vi "CommsTests.vi"() -> (2 "Pressure(hPa)":dbl format="%.1f")   [LabVIEW 2018]
uses:
  <vilib>/httpClient/LabVIEWHTTPClient.lvlib
panel:
  in  "timeout ms (60000)":i32=2000
  out "error out 2":errorcluster
  in  "remote port or service name":u16=2000
  in  "address":string="10.245.87.30"
  in  "data in":string="*SRHb\n"
  out "data out":string
  out "error out":errorcluster
  out "body":string
  out "headers":string="\r\n"
  in  "url":string="http://192.168.126.101"
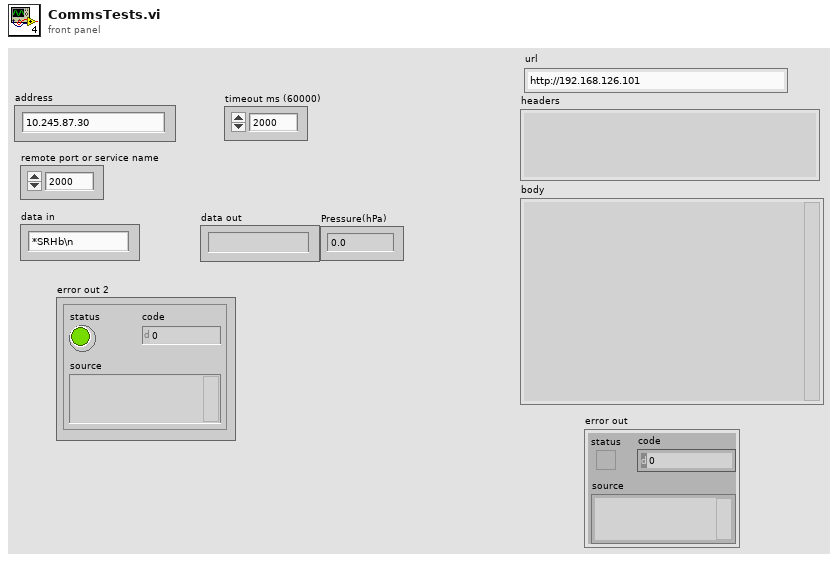
[diagram p1: front panel]
types:
  T1 = enum16{"Standard", "Buffered", "CRLF", "Immediate"}
  T2 = typedef "LabVIEWHTTPClient.lvlib/ClientHandle.ctl" = refnum<k1>
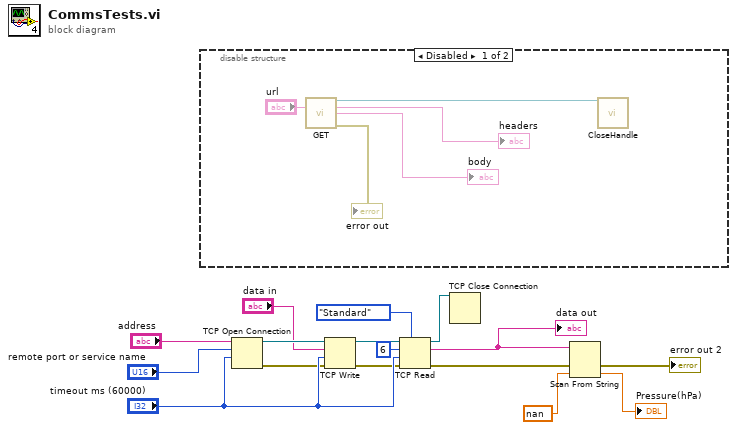
[diagram p0: block diagram]
diagram:
  n1 = disable-structure shown="Disabled" {
    frame Disabled {
      n2 = call <vilib>:"GET.vi"("url"="url") -> ("client handle out"=w17:T2, "headers"=→"headers":string, "body"=→"body":string, "error out"=→"error out":errorcluster)  [unwired: 11 in]
      n3 = call <vilib>:"CloseHandle.vi"("client handle"=w17) -> ()  [unwired: 14 in, 1 out]
    }
    frame Enabled {
    }
  }
  n4 = TCP Open Connection(address="address", remote port or service name="remote port or service name", timeout ms (60000)="timeout ms (60000)") -> (connection ID=w16:refnum<k5>, error out=w8:errorcluster)  [unwired: 2 in]
  n5 = TCP Write(connection ID=w16, data in="data in", error in (no error)=w8, 9:"timeout ms (60000)") -> (connection ID out=w15:refnum<k5>, error out=w7:errorcluster)  [unwired: 1 out]
  n6 = TCP Read(connection ID=w15, bytes to read=6, error in (no error)=w7, 7:T1."Standard" ("mode (standard)"), 9:"timeout ms (60000)") -> (connection ID out=w14:refnum<k5>, data out=w5:string, error out=w4:errorcluster)
  "data out" <- w5
  n7 = TCP Close Connection(connection ID=w14) -> ()  [unwired: 2 in, 2 out]
  n8 = Scan From String(input string=w5, error in=w4, default 1=nan ("default value 1")) -> (error out=→"error out 2":errorcluster, output 1=→"Pressure(hPa)":dbl)  [unwired: 2 in, 2 out]
